vi "CTRE_Phoenix_CANcoder_ConfigFeedbackCoefficient.vi"(0 "CTRE_CANcoder_DeviceRef":T2, 5 "sensorCoefficient":dbl, 7 "unitString":string, 9 "timebase":T1=enum."PerMinute", 11 "error in":errorcluster, 12 "timeoutMs":i32) -> (4 "CTRE_CANcoder_DeviceRef":T2, 15 "error out":errorcluster)   [LabVIEW 2019]
doc: "Choose what units you want the API to get/set. This also impacts the units displayed in Self-Test in Tuner. Depending on your mechanism, you may want to scale rotational units (deg, radians, rotations), or scale to a distance (inches, centimeters).\n\n<b>sensorCoefficient</b> Scalar to multiply the CANCoder's native 12-bit resolute sensor. Defaults to 0.087890625 to produce degrees.\n<b>unitString</b> String holding the unit to report in. This impacts all routines (except for ConfigMagnetOffset) and the self-test in Tuner. The string value itself is arbitrary. The max number of letters will depend on firmware versioning, but generally CANCoder supports up to eight letters. However, common units such as \"centimeters\" are supported explicitly despite exceeding the eight-letter limit. Default is \"deg\".\n<b>sensortimeBase</b> Desired denominator to report velocity in. This impacts GetVelocity and the reported velocity in self-test in Tuner. Default is \"Per Second\".\n<b>timeoutMs</b> Timeout value in ms. If nonzero, function will wait for config success and report an error if it times out. If zero, no blocking or checking is performed."
uses:
  <vilib>/Rock Robotics/WPI/ThirdParty/Phoenix-LabVIEW/CANCoder/Controls/CTRE_Phoenix_CANcoder_DeviceRef.ctl
  <vilib>/Rock Robotics/WPI/ThirdParty/Phoenix-LabVIEW/CANCoder/Controls/CTRE_Phoenix_CANcoder_SensorTimeBase.ctl
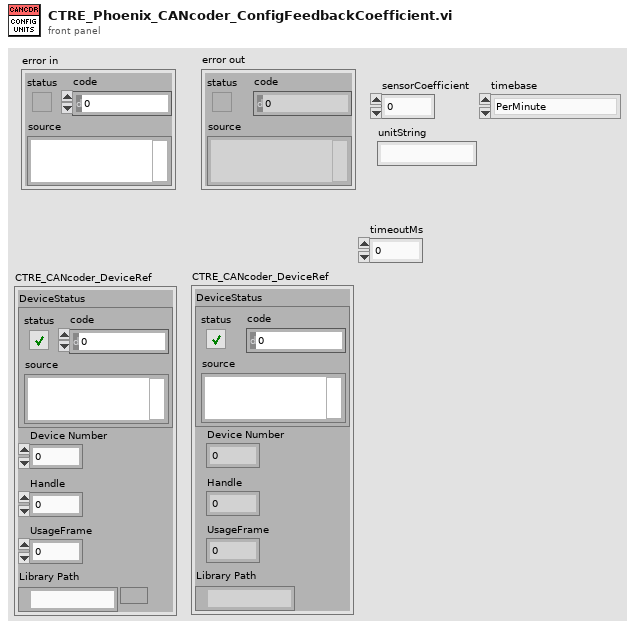
[diagram p1: front panel]
types:
  T1 = typedef "CTRE_Phoenix_CANcoder_SensorTimeBase.ctl" = enum16{"Per100Ms_Legacy", "PerSecond", "PerMinute"}
  T2 = typedef "CTRE_Phoenix_CANcoder_DeviceRef.ctl" = cluster{"DeviceStatus":errorcluster, "Device Number":u8, "Handle":u64, "UsageFrame":u32, "Library Path":path}
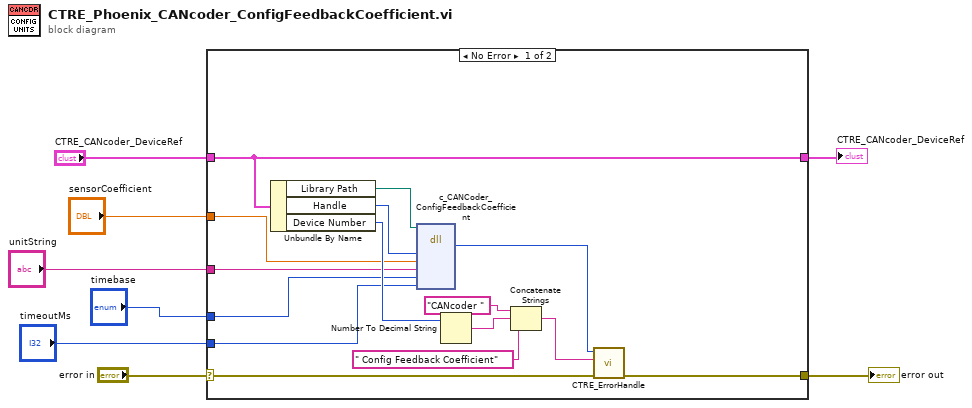
[diagram p0: block diagram]
diagram:
  n1 = case shown="No Error" "error in" {
    selector: "error in" -> [w20 w25]
    tunnel: "CTRE_CANcoder_DeviceRef" -> [w21 w24]
    tunnel: [w19 w25] -> w7
    tunnel: [w21 w24] -> w5
    tunnel: "sensorCoefficient" -> [w12 _]
    tunnel: "unitString" -> [w11 _]
    tunnel: "timebase" -> [w10 _]
    tunnel: "timeoutMs" -> [w9 _]
    frame No Error {
      n2 = Unbundle By Name(w21) -> ("Library Path"=w23:path, "Handle"=w22:u64, "Device Number"=w13:u8)
      n3 = dll-call lib="?" fn="c_CANCoder_ConfigFeedbackCoefficient"(path in=w23, "handle"=w22, "sensorCoefficient"=w12, "unitString"=w11, "timebase"=w10, "timeoutMs"=w9) -> ("CTR_Code"=w18:i8)  [unwired: 7 in, 2 out]
      n4 = Number To Decimal String(number=w13) -> (decimal integer string=w17:string)  [unwired: 1 in]
      n5 = Concatenate Strings("CANcoder " ("string"), w17, " Config Feedback Coefficient" ("string")) -> (w14:string)
      n6 = call <vilib>:"CTRE_ErrorHandle.vi"("error in"=w20, "origin"=w14, "code"=w18) -> ("error out"=w19:errorcluster)  [unwired: 8 in]
    }
    frame Error {
    }
  }
  "error out" <- w7
  "CTRE_CANcoder_DeviceRef" <- w5
